vi "Image (Mask) Characteristics.vi"(8 "error in (no error)":errorcluster, 10 "Image Mask Refnum":T1, 11 "Image Refnum":T1) -> (0 "error out":errorcluster, 3 "Mask ROI Statistics":T2, 4 "CPU (s)":dbl)   [LabVIEW 2021, in "Image.lvlib"]
uses:
  Image.lvlib
  Image ROI Statistics.ctl
  <vilib>/Analysis/NI_AALBase.lvlib
  <vilib>/Analysis/baseanly.llb/Unimode.vi
  Time/Time.lvlib
  <userlib>/_OpenG.lib/array/array.llb/openg_array.lvlib
  Phasor/Phasor.lvlib
  <userlib>/_OpenG.lib/array/array.llb/Filter 1D Array (DBL)__ogtk.vi
  <vilib>/vision/Image Controls.llb/IMAQ Image.ctl
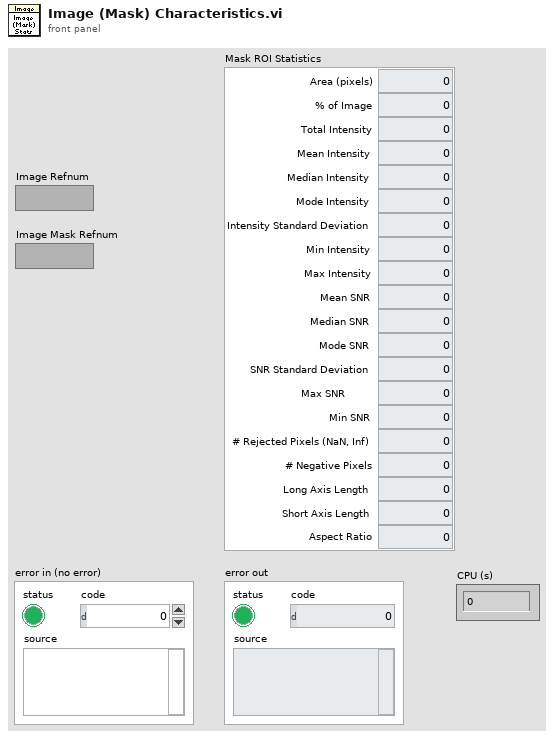
[diagram p1: front panel]
types:
  T1 = typedef "IMAQ Image.ctl" = refnum<image>
  T2 = typedef "Image.lvlib/Image ROI Statistics.ctl" = cluster{"Area (pixels)":dbl, "% of Image":dbl, "Total Intensity":dbl, "Mean Intensity":dbl, "Median Intensity":dbl, "Mode Intensity":dbl, "Intensity Standard Deviation":dbl, "Min Intensity":dbl, "Max Intensity":dbl, "Mean SNR":dbl, "Median SNR":dbl, "Mode SNR":dbl, "SNR Standard Deviation":dbl, "Max SNR":dbl, "Min SNR":dbl, "# Rejected Pixels (NaN, Inf)":dbl, "# Negative Pixels":dbl, "Long Axis Length":dbl, "Short Axis Length":dbl, "Aspect Ratio":dbl}
  T3 = typedef "Image.lvlib/Image Point.ctl" = cluster{"X":i32, "Y":i32}
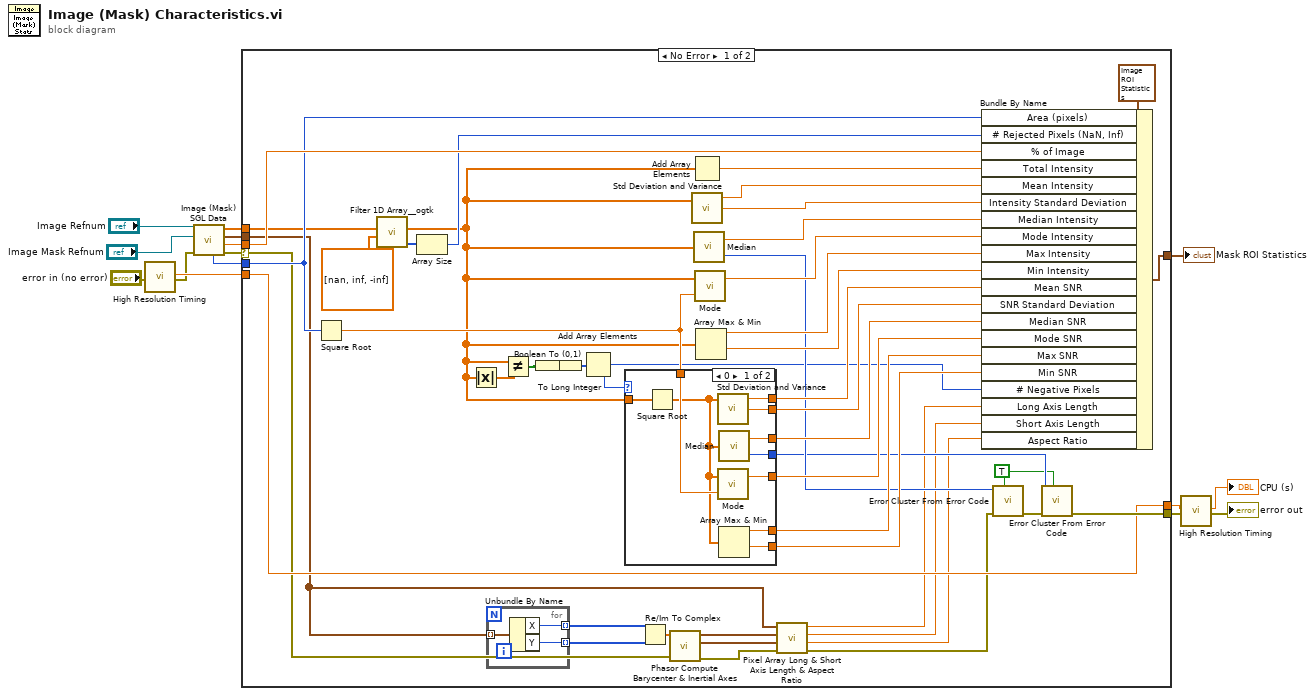
[diagram p0: block diagram]
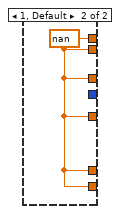
[diagram p2: hidden frame]
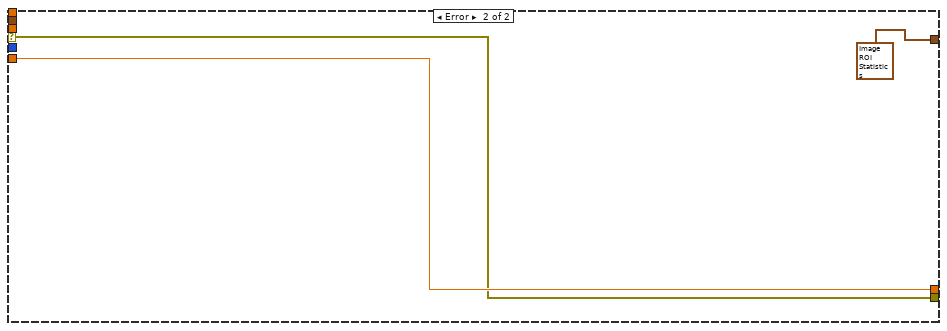
[diagram p3: hidden frame]
diagram:
  n1 = call "High Resolution Timing.vi"("Error In"="error in (no error)") -> ("elapsed (relative) seconds"=w11:dbl, "Error Out"=w6:errorcluster)  [unwired: 16 in, 1 out]
  n2 = call "Image (Mask) SGL Data.vi"("error in (no error)"=w6, "Image Mask Refnum"="Image Mask Refnum", "Src Image Refnum"="Image Refnum") -> ("error out"=w5:errorcluster, "% of Image"=w2:dbl, "[Pixel Coordinates]"=w3:T3[], "Pixel Values (SGL)"=w4:sgl[], "# Mask Pixels"=w1:i32)  [unwired: 3 in, 1 out]
  n3 = case shown="No Error" w5 {
    selector: w5 -> [w24 w76]
    tunnel: [w61 T2 {"Area (pixels)"=0.0, "% of Image"=0.0, "Total Intensity"=0.0, "Mean Intensity"=0.0, "Median Intensity"=0.0, "Mode Intensity"=0.0, "Intensity Standard Deviation"=0.0, "Min Intensity"=0.0, "Max Intensity"=0.0, "Mean SNR"=0.0, "Median SNR"=0.0, "Mode SNR"=0.0, "SNR Standard Deviation"=0.0, "Max SNR"=0.0, "Min SNR"=0.0, "# Rejected Pixels (NaN, Inf)"=0.0, "# Negative Pixels"=0.0, "Long Axis Length"=0.0, "Short Axis Length"=0.0, "Aspect Ratio"=0.0} ("ROI Statistics")] -> w15
    tunnel: [w42 w76] -> w13
    tunnel: [w41 w78] -> w10
    tunnel: w11 -> [w41 w78]
    tunnel: w4 -> [w36 _]
    tunnel: w3 -> [w23 _]
    tunnel: w2 -> [w38 _]
    tunnel: w1 -> [w37 _]
    frame No Error {
      w39 = TRUE ("show call chain? (False)")
      n4 = Square Root(x=w37) -> (sqrt(x)=w46:dbl)
      n5 = call-poly <userlib>:"Filter 1D Array__ogtk.vi"("items to filter"=dbl[] [nan, inf, -inf] ("Element(s) to Remove"), "array"=w36) -> ("filtered item indices"=w35:i32[], "filtered array"=w32:dbl[])  [unwired: 4 in]
      n6 = Array Size(array=w35) -> (size(s)=w34:i32)
      n7 = Absolute Value(x=w32) -> (abs(x)=w33:dbl[])
      n8 = for {
        tunnel: w23 -> [w64] mode=indexing
        tunnel: [w63] -> w27 mode=indexing
        tunnel: [w62] -> w26 mode=indexing
        n9 = Unbundle By Name(w64) -> ("X"=w63:i32, "Y"=w62:i32)
      }
      n10 = Not Equal?(x=w32, y=w33) -> (x != y?=w31:bool[])
      n11 = Boolean To (0,1)(Boolean=w31) -> (0, 1=w30:i16[])
      n12 = To Long Integer(number=w30) -> (32bit integer=w29:i32[])
      n13 = Add Array Elements(numeric array=w29) -> (sum=w28:i32)
      n14 = case shown="0" w28 {
        tunnel: [w74 w75] -> w52
        tunnel: [w73 w75] -> w51
        tunnel: [w72 w75] -> w50
        tunnel: [w71 w75] -> w49
        tunnel: [w70 w75] -> w48
        tunnel: [w69 w75] -> w47
        tunnel: w46 -> [w68 _]
        tunnel: [w67 _] -> w44
        tunnel: w32 -> [w65 _]
        frame 0 {
          n15 = Square Root(x=w65) -> (sqrt(x)=w66:dbl[])
          n16 = call <vilib>:"Std Deviation and Variance.vi"("X"=w66) -> ("mean"=w74:dbl, "standard deviation"=w73:dbl)  [unwired: 1 in, 1 out]
          n17 = call-poly <vilib>:"Mode.vi"("intervals"=w68, "X"=w66) -> ("mode"=w71:dbl)  [unwired: 1 out]
          n18 = call <vilib>:"Median.vi"("X"=w66) -> ("median"=w72:dbl, "error"=w67:i32)
          n19 = Array Max & Min(array=w66) -> (max value=w70:dbl, min value=w69:dbl)  [unwired: 2 out]
        }
        frame 1, Default {
          w75 = nan ("mean")
        }
      }
      n20 = Re/Im To Complex(1:w26, 2:w27) -> (0:w25:cdb[])
      n21 = call "Phasor Compute Barycenter & Inertial Axes.vi"("Error In"=w24, "Phasors"=w25) -> ("Error Out"=w20:errorcluster, "Major Axis"=w21:cluster{"x":dbl, "y":dbl}, "Barycenter"=w22:cluster{"x":sgl, "y":sgl})  [unwired: 5 in, 2 out]
      n22 = Add Array Elements(numeric array=w32) -> (sum=w53:dbl)
      n23 = call <vilib>:"Std Deviation and Variance.vi"("X"=w32) -> ("mean"=w59:dbl, "standard deviation"=w58:dbl)  [unwired: 1 in, 1 out]
      n24 = call <vilib>:"Median.vi"("X"=w32) -> ("median"=w57:dbl, "error"=w45:i32)
      n25 = call-poly <vilib>:"Mode.vi"("intervals"=w46, "X"=w32) -> ("mode"=w56:dbl)  [unwired: 1 out]
      n26 = Array Max & Min(array=w32) -> (max value=w55:dbl, min value=w54:dbl)  [unwired: 2 out]
      n27 = call "Pixel Array Long & Short Axis Length & Aspect Ratio.vi"("error in (no error)"=w20, "Direction"=w21, "Center"=w22, "Pixel Coordinates"=w23) -> ("error out"=w19:errorcluster, "Aspect Ratio"=w16:dbl, "Short Axis Length"=w17:dbl, "Long Axis Length"=w18:dbl)  [unwired: 4 in]
      n28 = Bundle By Name(cluster=T2 {"Area (pixels)"=0.0, "% of Image"=0.0, "Total Intensity"=0.0, "Mean Intensity"=0.0, "Median Intensity"=0.0, "Mode Intensity"=0.0, "Intensity Standard Deviation"=0.0, "Min Intensity"=0.0, "Max Intensity"=0.0, "Mean SNR"=0.0, "Median SNR"=0.0, "Mode SNR"=0.0, "SNR Standard Deviation"=0.0, "Max SNR"=0.0, "Min SNR"=0.0, "# Rejected Pixels (NaN, Inf)"=0.0, "# Negative Pixels"=0.0, "Long Axis Length"=0.0, "Short Axis Length"=0.0, "Aspect Ratio"=0.0} ("ROI Statistics"), "Area (pixels)"=w37, "# Rejected Pixels (NaN, Inf)"=w34, "% of Image"=w38, "Total Intensity"=w53, "Mean Intensity"=w59, "Intensity Standard Deviation"=w58, "Median Intensity"=w57, "Mode Intensity"=w56, "Max Intensity"=w55, "Min Intensity"=w54, "Mean SNR"=w52, "SNR Standard Deviation"=w51, "Median SNR"=w50, "Mode SNR"=w49, "Max SNR"=w48, "Min SNR"=w47, "# Negative Pixels"=w28, "Long Axis Length"=w18, "Short Axis Length"=w17, "Aspect Ratio"=w16) -> (w61:T2)
      n29 = call <vilib>:"Error Cluster From Error Code.vi"("show call chain? (False)"=w39, "error in (no error)"=w19, "error code (0)"=w45) -> ("error out"=w43:errorcluster)  [unwired: 6 in]
      n30 = call <vilib>:"Error Cluster From Error Code.vi"("show call chain? (False)"=w39, "error in (no error)"=w43, "error code (0)"=w44) -> ("error out"=w42:errorcluster)  [unwired: 6 in]
    }
    frame Error {
    }
  }
  "Mask ROI Statistics" <- w15
  n31 = call "High Resolution Timing.vi"("relative seconds (NaN)"=w10, "Error In"=w13) -> ("elapsed (relative) seconds"=→"CPU (s)":dbl, "Error Out"=→"error out":errorcluster)  [unwired: 15 in, 1 out]
